vi "Generate Struct Strings.vi"(8 "error in":errorcluster, 11 "Test Names":string) -> (0 "Error Out":errorcluster, 1 "Vendor ID":string="Cal Struct Set Strings_VendorID", 2 "Mfg Location":string="Cal Struct Set Strings_Mfg Location", 3 "PCB Assy No":string="Cal Struct Set Strings_PcbAssyNum", 4 "Mfr Date":string, 5 "PCB Rev":string="Cal Struct Set Strings_PcbRevision")   [LabVIEW 2013]
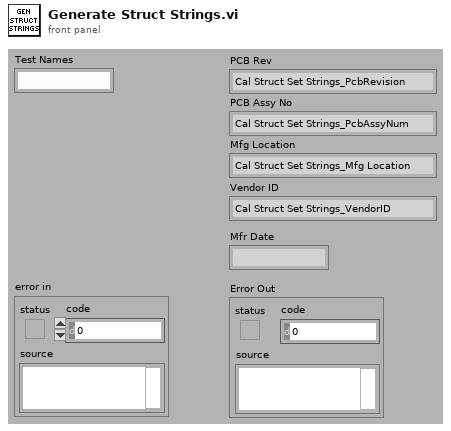
[diagram p1: front panel]
types:
  T1 = typedef "LVDateTimeRec.ctl" = cluster{"fractional second":dbl, "second":i32, "minute":i32, "hour":i32, "day of month":i32, "month":i32, "year":i32, "day of week":i32, "day of year":i32, "DST":i32}
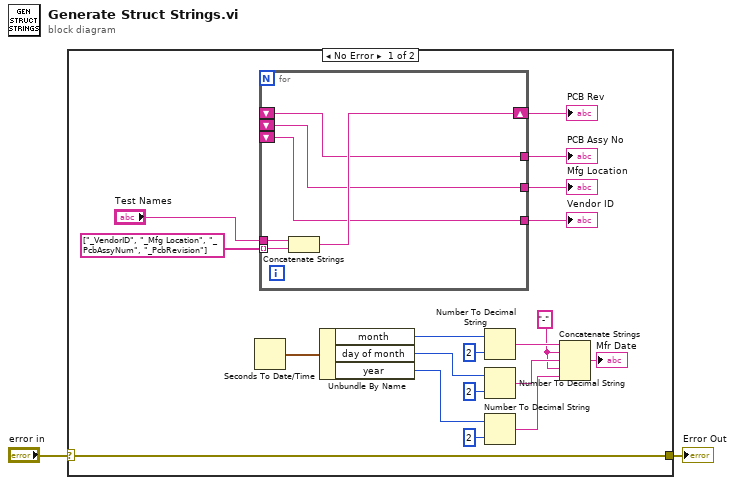
[diagram p0: block diagram]
diagram:
  n1 = case shown="No Error" "error in" {
    selector: "error in" -> [w3 w28]
    tunnel: [w3 w28] -> w1
    frame No Error {
      w7 = "-"
      n2 = Seconds To Date/Time() -> (date time rec=w16:T1)  [unwired: 2 in]
      n3 = for {
        tunnel: string[] ["_VendorID", "_Mfg Location", "_PcbAssyNum", "_PcbRevision"] -> [w27] mode=indexing
        tunnel: [w25] -> w19
        tunnel: [w24] -> w18
        tunnel: [w23] -> w17
        shift-right: [w26] -> w20
        shift-left: _ -> [w25]
        shift-left: _ -> [w24]
        shift-left: _ -> [w23]
        tunnel: "Test Names" -> [w22]
        n4 = Concatenate Strings(w22, w27) -> (w26:string)
      }
      "PCB Rev" <- w20
      "PCB Assy No" <- w19
      "Mfg Location" <- w18
      "Vendor ID" <- w17
      n5 = Unbundle By Name(w16) -> ("month"=w15:i32, "day of month"=w11:i32, "year"=w10:i32)
      n6 = Number To Decimal String(number=w15, width (-)=i16 2) -> (decimal integer string=w9:string)
      n7 = Number To Decimal String(number=w11, width (-)=i16 2) -> (decimal integer string=w8:string)
      n8 = Number To Decimal String(number=w10, width (-)=i16 2) -> (decimal integer string=w6:string)
      n9 = Concatenate Strings(w9, w7, w8, w7, w6) -> (→"Mfr Date":string)
    }
    frame Error {
    }
  }
  "Error Out" <- w1
